vi "comms loop main.vi"(11 "comms":T1) -> ()   [LabVIEW 2018]
uses:
  type defs/comms loop data.ctl
  ICL-LabVIEW_General/Incident logger/Incident logger.lvclass
  <vilib>/Modbus/master/Modbus Master.lvclass
  <vilib>/Utility/error.llb/DialogType.ctl
  ICL-LabVIEW_General/Message Scheduler/generic message queue/standard message queue/standard message.lvclass
  C:/GitHub/ICL-LabVIEW_General/Message Scheduler/generic message queue/generic message.lvclass
  ICL-LabVIEW_General/Incident logger/Incidents/Warning/Warning.lvclass
  C:/GitHub/ICL-LabVIEW_General/Incident logger/Incidents/Incident.lvclass
  ICL-LabVIEW_General/Incident logger/Incidents/Error/Error.lvclass
  supporting VIs/polymorphic VIs/de-queue for comms.vi
  ICL-LabVIEW_General/Pulser Controller/AKD MODBUS commands/home.vi
  supporting VIs/polymorphic VIs/release comms queue.vi
  ICL-LabVIEW_General/Message Scheduler/message scheduler.lvclass
  ICL-LabVIEW_General/Message Scheduler/scheduled message/scheduled message.lvclass
  ICL-LabVIEW_General/Pulser Controller/Pulser controller commands library.lvlib
types:
  T1 = typedef "comms loop data.ctl" = cluster{"params":cluster{"commandStream":cluster{"reader name":string, "writer name":string, "stream buffer size":i32}, "errorStream":cluster{"reader name":string, "writer name":string, "stream buffer size":i32}, "RT IP address":string, "pulserControllerIP":string}, "vars":cluster{"commandStream":refnum<k21>, "Incident logger":refnum<class "Incident logger.lvclass">, "check error scheduled message":u32, "errorStream":refnum<k21>, "watchdogScheduleID":u32, "pulsator":cluster{"pulser connection":refnum<class "Modbus Master.lvclass">, "pulserConnected":bool, "pulsatorScheduleID":u32, "pulserRunning":bool}}}
  T2 = typedef "Queues.ctl" = cluster{"messageHandler":refnum<queue>, "comms":refnum<queue>, "dataStream":refnum<queue>, "dataProcessor":refnum<queue>, "fileIO":refnum<queue>, "userInterface":refnum<queue>, "errors":refnum<queue>, "customCompressor":refnum<queue>}
  T3 = cluster{"Target":string, "Loop":string, "Code":string}
  T4 = cluster{"standard message out":refnum<class "standard message.lvclass">, "ms delay":u32}
  T5 = typedef "DialogType.ctl" = u16
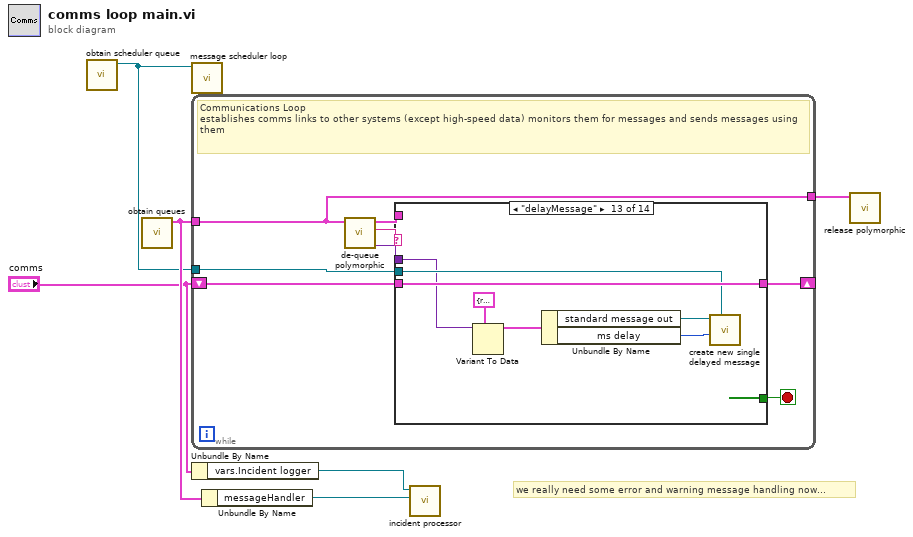
[diagram p0: block diagram]
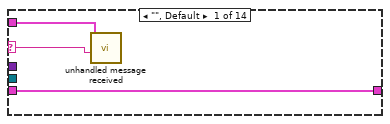
[diagram p2: hidden frame]
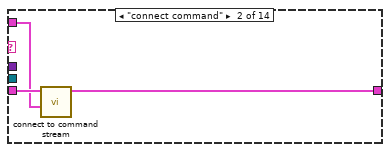
[diagram p3: hidden frame]
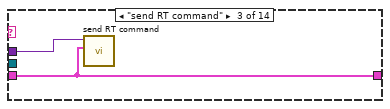
[diagram p4: hidden frame]
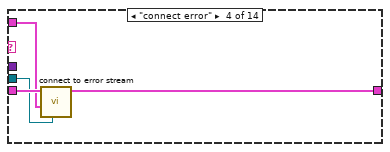
[diagram p5: hidden frame]
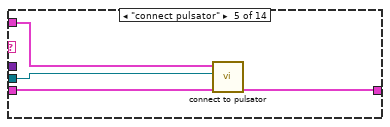
[diagram p6: hidden frame]
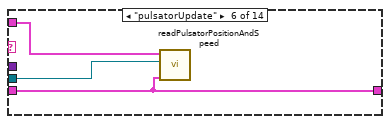
[diagram p7: hidden frame]
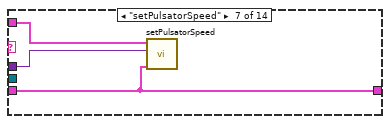
[diagram p8: hidden frame]
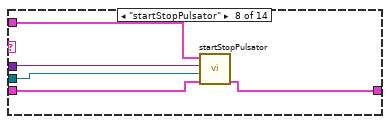
[diagram p9: hidden frame]
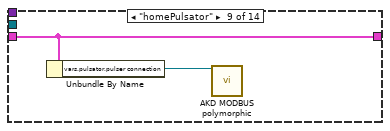
[diagram p10: hidden frame]
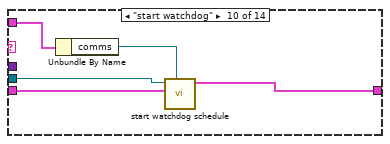
[diagram p11: hidden frame]
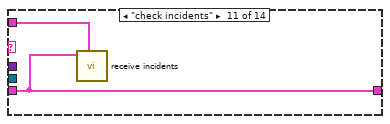
[diagram p12: hidden frame]
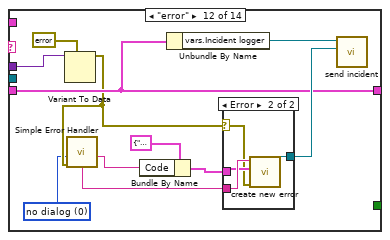
[diagram p13: hidden frame]
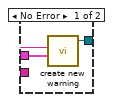
[diagram p14: hidden frame]
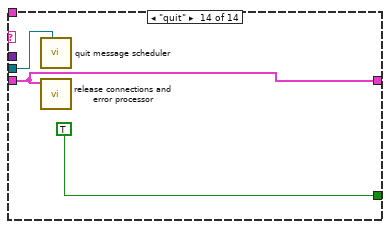
[diagram p15: hidden frame]
diagram:
  # "we really need some error and warning message handling now..."
  n1 = call "obtain scheduler queue.vi"() -> ("message scheduler out"=w2:refnum<class "message scheduler.lvclass">)  [unwired: 10 in, 1 out]
  n2 = call "obtain queues.vi"() -> ("queues"=w6:T2)  [unwired: 11 in]
  n3 = call "message scheduler loop.vi"("message scheduler"=w2) -> ()  [unwired: 11 in]
  n4 = while {
    tunnel: w6 -> [w7]
    tunnel: w2 -> [w10]
    shift-right: [w9] -> _
    shift-left: "comms" -> [w8]
    tunnel: [w7] -> w3
    stop <- w12 stop-if-true
    # "Communications Loop\nestablishes comms links to other systems (except high-speed data) monitors them for messages and sends messages using them"
    n5 = call-poly "de-queue polymorphic.vi"("Queues"=w7) -> ("data"=w13:variant, "message"=w14:string, "Queues out"=w11:T2)  [unwired: 8 in]
    n6 = case shown="\"delayMessage\"" w14 {
      selector: w14 -> [w15 _ _ _ _ _ _ _ _ _ _ _ _ _]
      tunnel: w13 -> [_ _ w22 _ _ _ w35 w40 _ _ _ w58 w73 _]
      tunnel: [_ _ _ _ _ _ _ _ _ _ _ _ _ TRUE] -> w12
      tunnel: w11 -> [w16 w18 _ w23 w30 w33 w36 w41 _ w45 w49 _ _ _]
      tunnel: w10 -> [_ _ _ w24 w27 w31 _ w38 _ w46 _ _ w74 w76]
      tunnel: [w17 w19 w21 w26 w28 w32 w34 w37 w43 w47 w50 w60 w75 w77] -> w9
      tunnel: w8 -> [w17 w20 w21 w25 w29 w32 w34 w39 w43 w48 w50 w60 w75 w77]
      frame "", Default {
        n7 = call "unhandled message received.vi"("unhandledMessage"=w15, "queues"=w16) -> ()  [unwired: 10 in]
      }
      frame "connect command" {
        n8 = call "connect to command stream.vi"("Queues"=w18, "comms in"=w20) -> ("comms out"=w19:T1)  [unwired: 9 in]
      }
      frame "send RT command" {
        n9 = call "send RT command.vi"("comms in"=w21, "data"=w22) -> ()  [unwired: 9 in, 1 out]
      }
      frame "connect error" {
        n10 = call "connect to error stream.vi"("message scheduler"=w24, "Queues"=w23, "comms in"=w25) -> ("comms out"=w26:T1)  [unwired: 8 in]
      }
      frame "connect pulsator" {
        n11 = call "connect to pulsator.vi"("comms in"=w29, "message scheduler"=w27, "queues"=w30) -> ("comms out"=w28:T1)  [unwired: 8 in]
      }
      frame "pulsatorUpdate" {
        n12 = call "readPulsatorPositionAndSpeed.vi"("comms"=w32, "message scheduler"=w31, "Queues"=w33) -> ()  [unwired: 9 in]
      }
      frame "setPulsatorSpeed" {
        n13 = call "setPulsatorSpeed.vi"("comms"=w34, "speed data"=w35, "Queues"=w36) -> ()  [unwired: 9 in]
      }
      frame "startStopPulsator" {
        n14 = call "startStopPulsator.vi"("comms"=w39, "message scheduler"=w38, "start?"=w40, "Queues"=w41) -> ("comms out"=w37:T1)  [unwired: 7 in]
      }
      frame "homePulsator" {
        n15 = Unbundle By Name(w43) -> ("vars.pulsator.pulser connection"=w42:refnum<class "Modbus Master.lvclass">)
        n16 = call-poly "AKD MODBUS polymorphic.vi"("Modbus Master in"=w42) -> ()  [unwired: 10 in, 1 out]
      }
      frame "start watchdog" {
        n17 = Unbundle By Name(w45) -> ("comms"=w44:refnum<queue>)
        n18 = call "start watchdog schedule.vi"("comms queue"=w44, "comms in"=w48, "message scheduler in"=w46) -> ("comms out"=w47:T1)  [unwired: 8 in]
      }
      frame "check incidents" {
        n19 = call "receive incidents.vi"("queues"=w49, "comms in"=w50) -> ()  [unwired: 10 in]
      }
      frame "error" {
        w51 = T5 0 items=["no dialog", "OK message", "continue or stop message", "OK message + warnings", "continue/stop + warnings"] ("type of dialog (OK msg:1)")
        n20 = Variant To Data(type=errorcluster {"status"=FALSE, "code"=0, "source"=""} ("error constant"), Variant=w58) -> (data=w55:errorcluster)  [unwired: 1 in, 1 out]
        n21 = call <vilib>:"Simple Error Handler.vi"("type of dialog (OK msg:1)"=w51, "error in (no error)"=w55) -> ("source out"=w52:string, "message"=w56:string)  [unwired: 3 in, 3 out]
        n22 = Bundle By Name(cluster=T3 {"Target"="PC", "Loop"="", "Code"=""} ("Location"), "Code"=w52) -> (w53:T3)
        n23 = Unbundle By Name(w60) -> ("vars.Incident logger"=w59:refnum<class "Incident logger.lvclass">)
        n24 = case shown="Error" w55 {
          selector: w55 -> [_ w65]
          tunnel: [w64 w68] -> w61
          tunnel: w56 -> [w63 w67]
          tunnel: w53 -> [w62 w66]
          frame No Error {
            n25 = call "create new warning.vi"("Location"=w62, "Description"=w63) -> ("Warning out"=w64:refnum<class "Warning.lvclass">)  [unwired: 8 in, 1 out]
          }
          frame Error {
            n26 = call "create new error.vi"("Error"=w65, "Location"=w66, "Description"=w67) -> ("created error"=w68:refnum<class "Error.lvclass">)  [unwired: 8 in]
          }
        }
        n27 = call "send incident.vi"("incident"=w61, "Incident logger in"=w59) -> ()  [unwired: 8 in, 2 out]
      }
      frame "delayMessage" {
        n28 = Variant To Data(type=T4 {"standard message out"=refnum, "ms delay"=1000}, Variant=w73) -> (data=w71:T4)  [unwired: 1 in, 1 out]
        n29 = Unbundle By Name(w71) -> ("standard message out"=w70:refnum<class "standard message.lvclass">, "ms delay"=w69:u32)
        n30 = call "create new single delayed message.vi"("message scheduler"=w74, "ms delay"=w69, "generic message queue.lvclass"=w70) -> ()  [unwired: 8 in, 1 out]
      }
      frame "quit" {
        n31 = call "quit message scheduler.vi"("message scheduler"=w76) -> ()  [unwired: 10 in, 1 out]
        n32 = call "release connections and error processor.vi"("comms"=w77) -> ()  [unwired: 11 in]
      }
    }
  }
  n33 = Unbundle By Name("comms") -> ("vars.Incident logger"=w1:refnum<class "Incident logger.lvclass">)
  n34 = Unbundle By Name(w6) -> ("messageHandler"=w5:refnum<queue>)
  n35 = call "incident processor.vi"("message queue"=w5, "Incident logger in"=w1) -> ()  [unwired: 10 in]
  n36 = call-poly "release polymorphic.vi"("Queues"=w3) -> ()  [unwired: 11 in]
